vi "Default Configuration Reader.vi"(11 "Zone Setup Array ref":refnum<vi>) -> ()   [LabVIEW 2025]
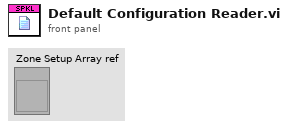
[diagram p1: front panel]
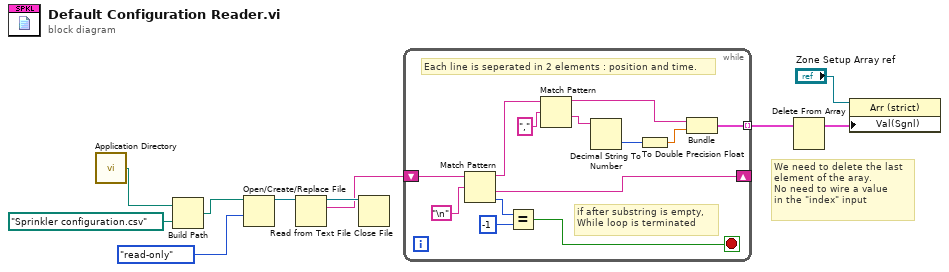
[diagram p0: block diagram]
diagram:
  # "We need to delete the last \nelement of the aray.\nNo need to wire a value\nin the \"index\" input"
  n1 = call <vilib>:"Application Directory.vi"() -> ("Application Directory"=w10:path)
  n2 = Build Path(base path=w10, name or relative path=path "Sprinkler configuration.csv") -> (appended path=w8:path)
  n3 = Open/Create/Replace File(file path (use dialog)=w8, access (0:read/write)=enum16{"read/write", "read-only", "write-only"}."read-only") -> (refnum out=w6:refnum<file>)  [unwired: 4 in, 2 out]
  n4 = Read from Text File(file (use dialog)=w6) -> (refnum out=w5:refnum<file>, text=w4:string)  [unwired: 3 in, 2 out]
  n5 = Close File(refnum=w5) -> ()  [unwired: 1 in, 2 out]
  n6 = while {
    shift-right: [w21] -> _
    shift-left: w4 -> [w23]
    tunnel: [w11] -> w3 mode=indexing
    stop <- w18 stop-if-true
    # "Each line is seperated in 2 elements : position and time."
    # "if after substring is empty, \nWhile loop is terminated"
    n7 = Match Pattern(string=w23, regular expression="\n") -> (before substring=w17:string, after substring=w21:string, offset past match=w20:i32)  [unwired: 1 in, 1 out]
    n8 = Equal?(x=w20, y=-1) -> (x = y?=w18:bool)
    n9 = Match Pattern(string=w17, regular expression=",") -> (before substring=w12:string, after substring=w15:string)  [unwired: 1 in, 2 out]
    n10 = Decimal String To Number(string=w15) -> (number=w14:i32)  [unwired: 2 in, 1 out]
    n11 = To Double Precision Float(number=w14) -> (double precision float=w13:dbl)
    n12 = Bundle(w12, w13) -> (w11:cluster{string, dbl})  [unwired: 1 in]
  }
  n13 = Delete From Array(array=w3) -> (array with subset deleted=w2:cluster{string, dbl}[])  [unwired: 2 in, 1 out]
  n14 = property class="Arr (strict)"(reference="Zone Setup Array ref", "Val(Sgnl)"=w2) -> ()  [unwired: 1 in, 2 out]
